vi "Pre Launch Init.vi"(11 "Nested in":refnum<class "Nested.lvclass">) -> (0 "error out":errorcluster, 3 "Nested out":refnum<class "Nested.lvclass">)   [LabVIEW 2025, in "Nested.lvlib" / "Nested.lvclass"]
doc: "(<B>Filename</B>: Actor Framework.lvlib:Actor.lvclass:Pre Launch Init.vi)\n\nDefines behavior that occurs after the Launch Nested Actor method is invoked but before the actor's Actor Core method begins running.\n\nBy default, this method does nothing. A descendant class may override it to define behavior."
uses:
  Nested.lvclass
  Nested.lvclass/Nested.ctl
  <vilib>/ActorFramework/Actor/Actor.lvclass
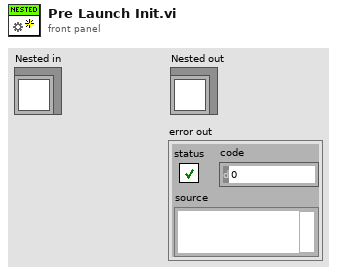
[diagram p1: front panel]
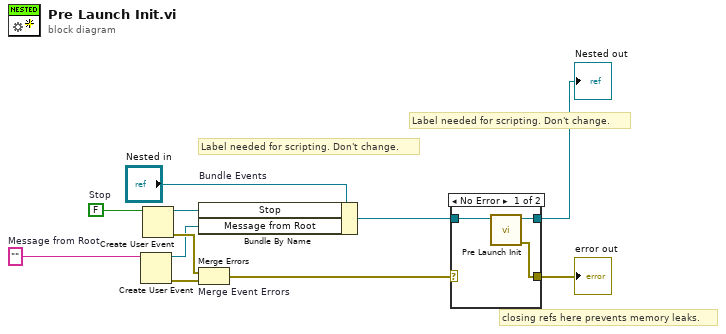
[diagram p0: block diagram]
diagram:
  w3 = ""  # Message from Root
  w10 = FALSE  # Stop
  # "Label needed for scripting. Don't change."
  # "Label needed for scripting. Don't change."
  # "closing refs here prevents memory leaks."
  n1 = Create User Event(user event datatype=w3) -> (user event=w2:refnum<user-event>, error out=w1:errorcluster)  [unwired: 1 in]
  n2 = Create User Event(user event datatype=w10) -> (user event=w8:refnum<user-event>, error out=w9:errorcluster)  [unwired: 1 in]
  n3 = Bundle By Name "Bundle Events"(cluster="Nested in", "Stop"=w8, "Message from Root"=w2) -> (w7:refnum<class "Nested.lvclass">)
  n4 = Merge Errors "Merge Event Errors"(w9, w1) -> (w6:errorcluster)
  n5 = case shown="No Error" w6 {
    selector: w6 -> [_ w16]
    tunnel: [w14 w15] -> w5
    tunnel: w7 -> [w13 w15]
    tunnel: [w12 w16] -> w4
    frame No Error {
      n6 = call-parent "Pre Launch Init.vi"("Actor in"=w13) -> ("error out"=w12:errorcluster, "Actor out"=w14:refnum<class "Nested.lvclass">)  [unwired: 9 in]
    }
    frame Error {
    }
  }
  "error out" <- w4
  "Nested out" <- w5
